vi "Handle LogRec.vi"(8 "error in":errorcluster, 10 "LogRecord":refnum<class "LogRecord.lvclass">, 11 "Handler in":refnum<class "Handler.lvclass">) -> (0 "error out":errorcluster, 3 "Handler out":refnum<class "Handler.lvclass">)   [LabVIEW 2020, in "hse-logger.lvlib" / "Handler.lvclass"]
doc: "Handles the incoming ``LogRecord`` object.\n\nThis method is the implementation of the base-class and does nothing. Use a pre-defined sub-class or implement your own.\n\n____\nHAMPEL SOFTWARE ENGINEERING v2.0.6 (2021-04-15 11:38)"
uses:
  Handler.lvclass
  LogRecord/LogRecord.lvclass
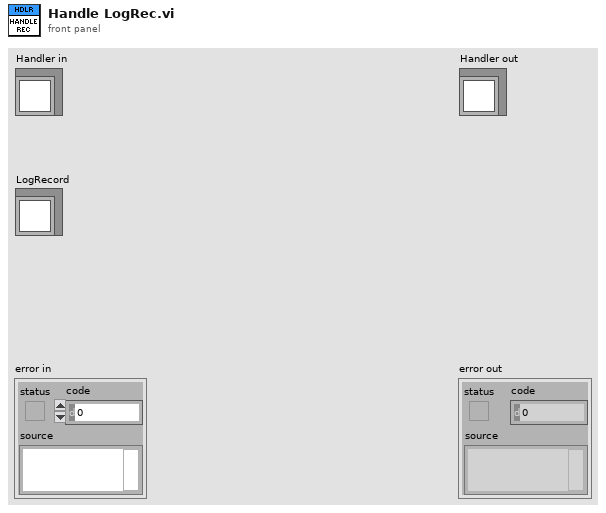
[diagram p1: front panel]
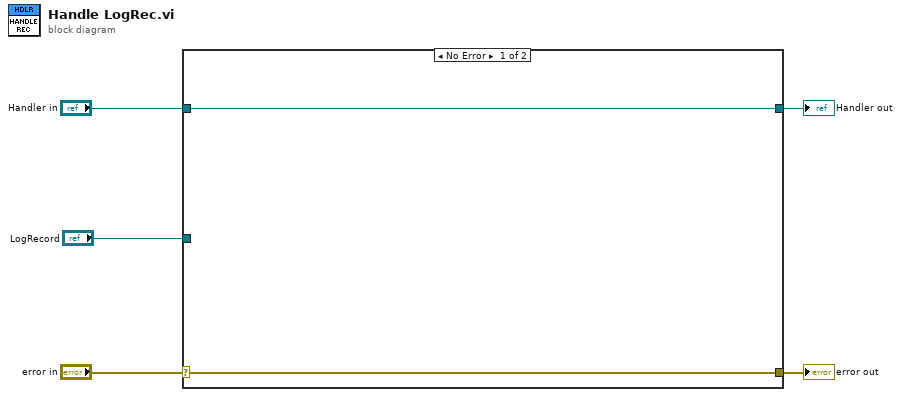
[diagram p0: block diagram]
diagram:
  n1 = case shown="No Error" "error in" {
    selector: "error in" -> [w6 w9]
    tunnel: [w6 w9] -> w4
    tunnel: [w7 w8] -> w2
    tunnel: "Handler in" -> [w7 w8]
    tunnel: "LogRecord" -> [_ _]
    frame No Error {
    }
    frame Error {
    }
  }
  "error out" <- w4
  "Handler out" <- w2
